vi "Find Item.vi"(7 "$Path or Item Name":string, 8 "error in (no error)":errorcluster, 10 "Offset":i32, 11 "JSON":string) -> (0 "error out":errorcluster, 1 "<JSON>":string caption="<JSON>Item", 2 "Item offset":i32, 3 "Found":bool)   [LabVIEW 2021, in "jsontext.facade.lvlib"]
doc: "Find the JSON item at the JSON Path specified.\n\nPaths specify an item in a tree of nested Objects, and start with $.\nExample JSON:\n{\"A\":{\"A1\":123,\"A2\":4},\"B\":\"Hi\"}\nAt path $.A.A1 is 123\nAt path $.B (or just B) is \"Hi\"\nAt path $.A (or just A) is {\"A1\":123,\"A2\":4}"
uses:
  jsontext.facade.lvlib
  jsontext/String Subset.vi
  jsontext/Parsing/Parse Full Path or Item Name.vi
  jsontext/Next JSON Value.vi
  jsontext/support/Error Cluster From Code.vi
  jsontext/Offset/Find Item Locations by Path.vi
  jsontext/JSONtext.lvlib
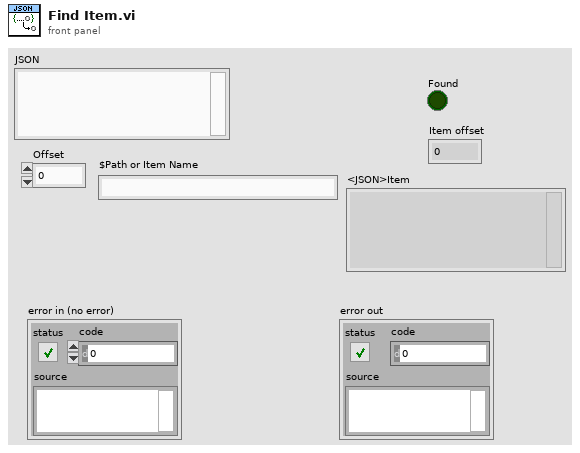
[diagram p1: front panel]
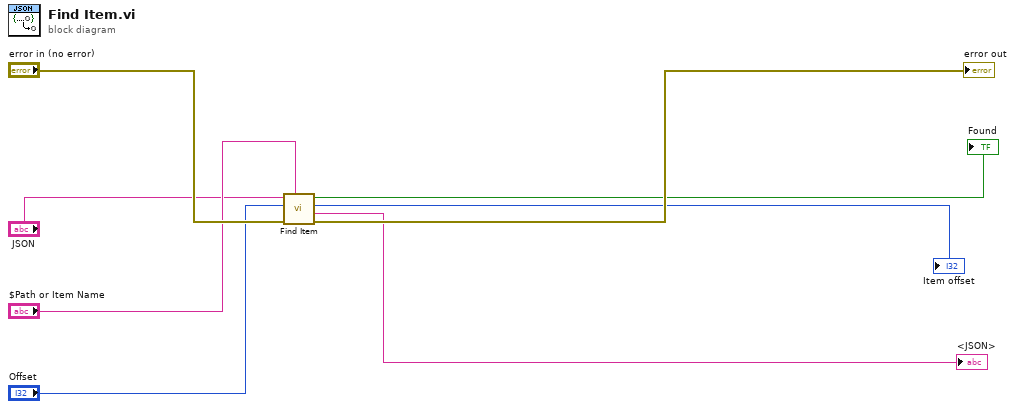
[diagram p0: block diagram]
diagram:
  n1 = call "Find Item.vi"("$Path or Item Name"="$Path or Item Name", "error in (no error)"="error in (no error)", "Offset"="Offset", "JSON"="JSON") -> ("error out"=→"error out":errorcluster, "<JSON>"=→"<JSON>":string, "Item offset"=→"Item offset":i32, "Found"=→"Found":bool)  [unwired: 4 in]
